vi "HostCriticalSection.vi"() -> ()   [LabVIEW 2014]
panel:
  out "Delta time":u32
  out "Result":i32
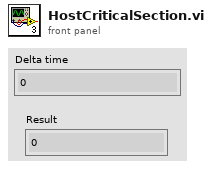
[diagram p1: front panel]
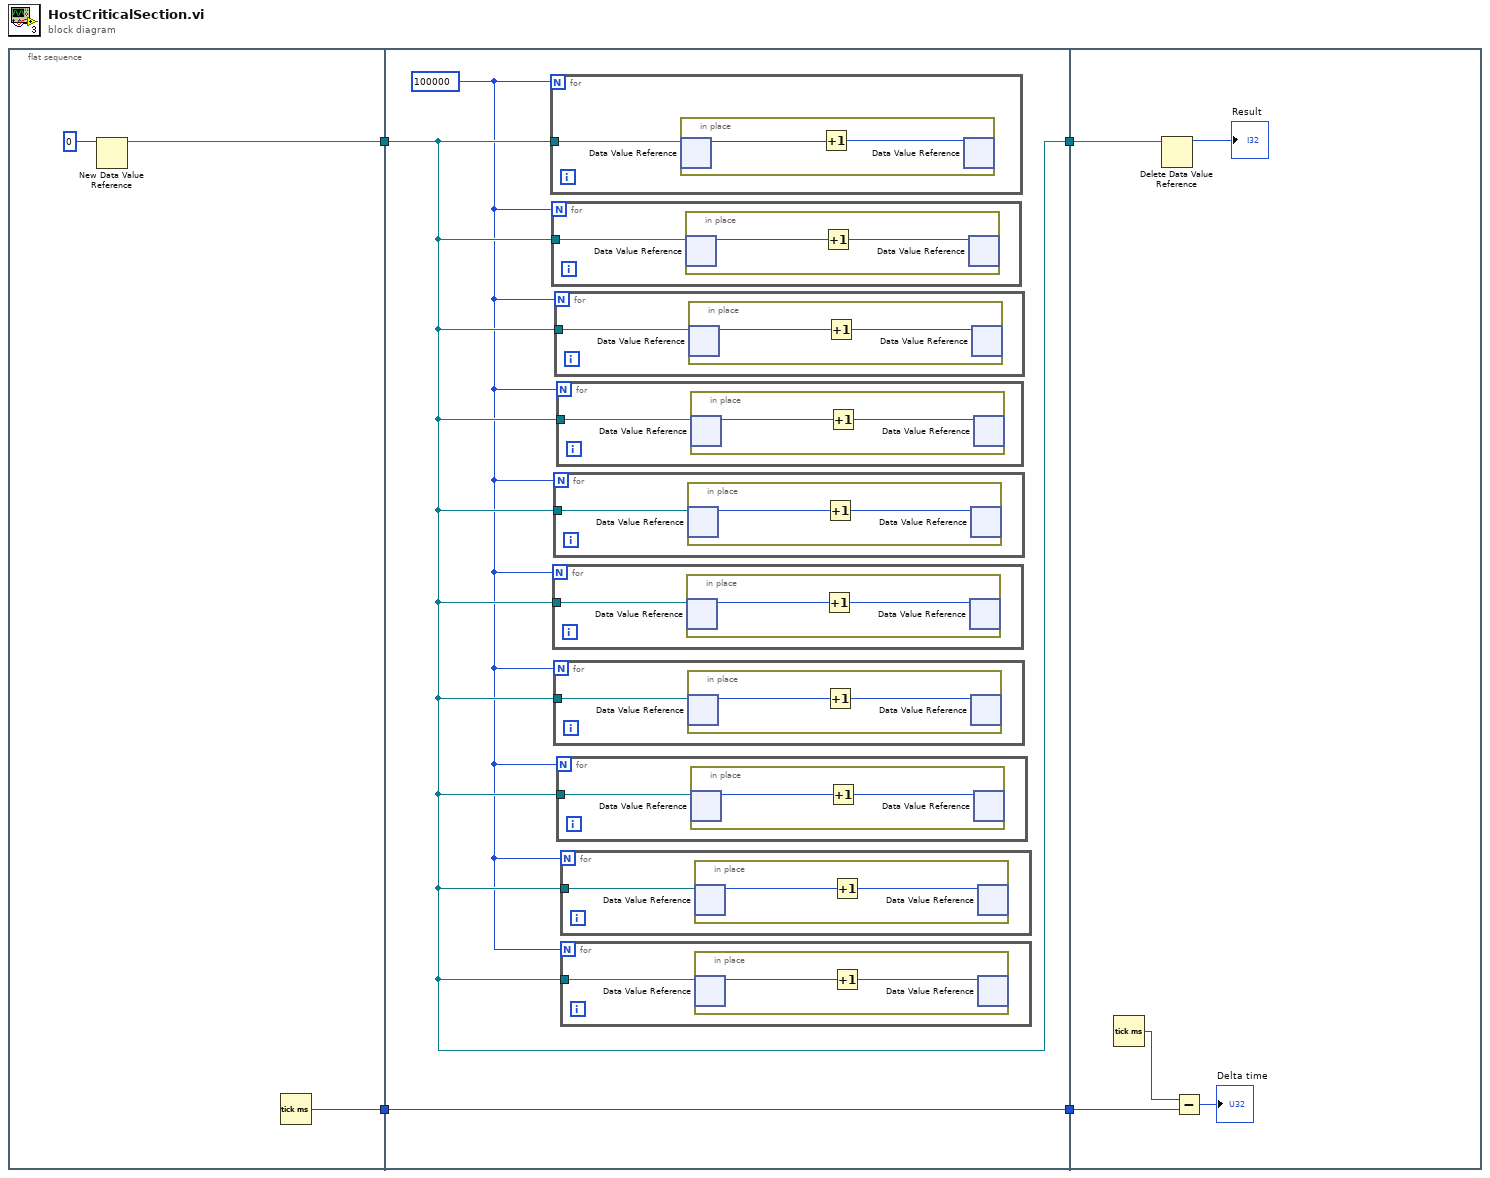
[diagram p0: block diagram]
diagram:
  n1 = flat-sequence {
    tunnel: [w6] -> w4
    tunnel: [w5] -> w2
    tunnel: w4 -> [w10]
    tunnel: [w10] -> w3
    tunnel: w2 -> [w9]
    tunnel: [w9] -> w1
    tunnel: w3 -> [w45]
    tunnel: w1 -> [w42]
    frame #0 {
      n2 = New Data Value Reference(data value=0) -> (data value reference=w6:refnum<data-value>)  [unwired: 1 in, 1 out]
      n3 = Tick Count (ms)() -> (millisecond timer value=w5:u32)
    }
    frame #1 {
      w8 = 100000
      n4 = for {
        N: w8 -> [_]
        tunnel: w10 -> [w38]
        n5 = in-place {
          n6 = in-place-dvr #1(w38) -> (w40:i32)  [unwired: 1 out]
          n7 = Increment(x=w40) -> (x+1=w39:i32)
          n8 = in-place-dvr #1(w39) -> ()  [unwired: 2 out]
        }
      }
      n9 = for {
        N: w8 -> [_]
        tunnel: w10 -> [w35]
        n10 = in-place {
          n11 = in-place-dvr #2(w35) -> (w37:i32)  [unwired: 1 out]
          n12 = Increment(x=w37) -> (x+1=w36:i32)
          n13 = in-place-dvr #2(w36) -> ()  [unwired: 2 out]
        }
      }
      n14 = for {
        N: w8 -> [_]
        tunnel: w10 -> [w23]
        n15 = in-place {
          n16 = in-place-dvr #3(w23) -> (w25:i32)  [unwired: 1 out]
          n17 = Increment(x=w25) -> (x+1=w24:i32)
          n18 = in-place-dvr #3(w24) -> ()  [unwired: 2 out]
        }
      }
      n19 = for {
        N: w8 -> [_]
        tunnel: w10 -> [w26]
        n20 = in-place {
          n21 = in-place-dvr #4(w26) -> (w28:i32)  [unwired: 1 out]
          n22 = Increment(x=w28) -> (x+1=w27:i32)
          n23 = in-place-dvr #4(w27) -> ()  [unwired: 2 out]
        }
      }
      n24 = for {
        N: w8 -> [_]
        tunnel: w10 -> [w20]
        n25 = in-place {
          n26 = in-place-dvr #5(w20) -> (w22:i32)  [unwired: 1 out]
          n27 = Increment(x=w22) -> (x+1=w21:i32)
          n28 = in-place-dvr #5(w21) -> ()  [unwired: 2 out]
        }
      }
      n29 = for {
        N: w8 -> [_]
        tunnel: w10 -> [w32]
        n30 = in-place {
          n31 = in-place-dvr #6(w32) -> (w34:i32)  [unwired: 1 out]
          n32 = Increment(x=w34) -> (x+1=w33:i32)
          n33 = in-place-dvr #6(w33) -> ()  [unwired: 2 out]
        }
      }
      n34 = for {
        N: w8 -> [_]
        tunnel: w10 -> [w29]
        n35 = in-place {
          n36 = in-place-dvr #7(w29) -> (w31:i32)  [unwired: 1 out]
          n37 = Increment(x=w31) -> (x+1=w30:i32)
          n38 = in-place-dvr #7(w30) -> ()  [unwired: 2 out]
        }
      }
      n39 = for {
        N: w8 -> [_]
        tunnel: w10 -> [w17]
        n40 = in-place {
          n41 = in-place-dvr #8(w17) -> (w19:i32)  [unwired: 1 out]
          n42 = Increment(x=w19) -> (x+1=w18:i32)
          n43 = in-place-dvr #8(w18) -> ()  [unwired: 2 out]
        }
      }
      n44 = for {
        N: w8 -> [_]
        tunnel: w10 -> [w14]
        n45 = in-place {
          n46 = in-place-dvr #9(w14) -> (w16:i32)  [unwired: 1 out]
          n47 = Increment(x=w16) -> (x+1=w15:i32)
          n48 = in-place-dvr #9(w15) -> ()  [unwired: 2 out]
        }
      }
      n49 = for {
        N: w8 -> [_]
        tunnel: w10 -> [w11]
        n50 = in-place {
          n51 = in-place-dvr #10(w11) -> (w13:i32)  [unwired: 1 out]
          n52 = Increment(x=w13) -> (x+1=w12:i32)
          n53 = in-place-dvr #10(w12) -> ()  [unwired: 2 out]
        }
      }
    }
    frame #2 {
      n54 = Tick Count (ms)() -> (millisecond timer value=w43:u32)
      n55 = Delete Data Value Reference(data value reference=w45) -> (data value=→"Result":i32)  [unwired: 1 in, 1 out]
      n56 = Subtract(x=w43, y=w42) -> (x-y=→"Delta time":u32)
    }
  }
